vi "Read Status.vi"(8 "error in (no error)":errorcluster, 11 "SimFlatShutt in":refnum<class "SimFlatShutt.lvclass">) -> (0 "error out":errorcluster, 2 "Status":bool, 3 "SimFlatShutt out":refnum<class "SimFlatShutt.lvclass">)   [LabVIEW 2016, in "SimFlatShutt.lvclass"]
uses:
  SimFlatShutt.lvclass
  Shutter.lvclass
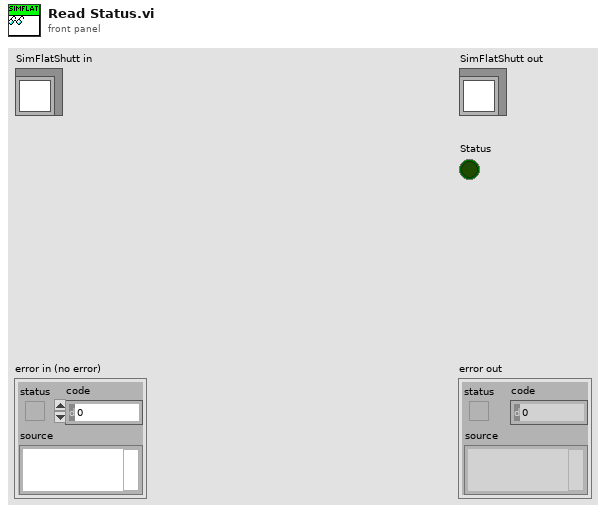
[diagram p1: front panel]
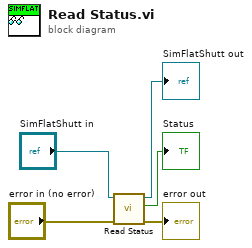
[diagram p0: block diagram]
diagram:
  n1 = call-parent "Read Status.vi"("error in (no error)"="error in (no error)", "Shutter in"="SimFlatShutt in") -> ("error out"=→"error out":errorcluster, "Status"=→"Status":bool, "Shutter out"=→"SimFlatShutt out":refnum<class "SimFlatShutt.lvclass">)  [unwired: 7 in]
